vi "FTW-Publisher-Publish.vi"(0 "FTW-Publisher In":refnum<class "FTW-Publisher.lvclass">, 5 "Header":string, 7 "Body":string, 11 "error in":errorcluster) -> (4 "FTW-Publisher Out":refnum<class "FTW-Publisher.lvclass">, 15 "error out":errorcluster)   [LabVIEW 2013, in "FTW-Publisher.lvclass"]
uses:
  FTW-Publisher.lvclass
  Message/Base/FTW-Message.lvclass
  FTW-Publisher.lvclass/FTW-Publisher.ctl
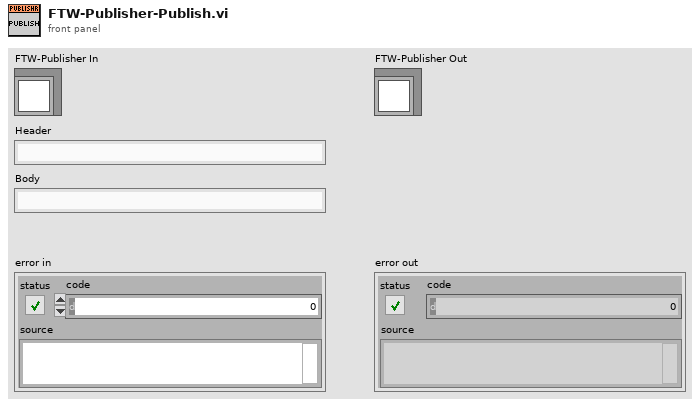
[diagram p1: front panel]
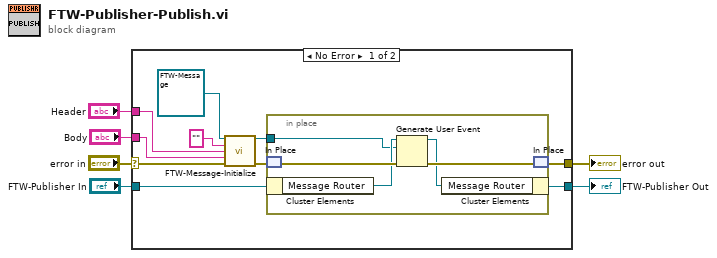
[diagram p0: block diagram]
diagram:
  n1 = case shown="No Error" "error in" {
    selector: "error in" -> [w14 w23]
    tunnel: [w13 w23] -> w3
    tunnel: [w15 w22] -> w5
    tunnel: "FTW-Publisher In" -> [w16 w22]
    tunnel: "Header" -> [w9 _]
    tunnel: "Body" -> [w8 _]
    frame No Error {
      n2 = call-dynamic "FTW-Message-Initialize.vi"("FTW Message"=refnum<class "FTW-Message.lvclass"> refnum, "Sender Identity"="", "Message Header"=w9, "Message Body"=w8, "error in"=w14) -> ("FTW Message out"=w11:refnum<class "FTW-Message.lvclass">, "error out"=w12:errorcluster)  [unwired: 9 in]
      n3 = in-place {
        in-place-border: w11 -> [w17]
        n4 = in-place-match #1(w12) -> (w21:errorcluster)
        n5 = in-place-cluster #2(w16) -> ("Message Router"=w20:refnum<user-event>)
        n6 = Generate User Event(user event=w20, event data cluster=w17, error in=w21) -> (user event out=w18:refnum<user-event>, error out=w19:errorcluster)  [unwired: 1 in]
        n7 = in-place-cluster #2("Message Router"=w18) -> (w15:refnum<class "FTW-Publisher.lvclass">)
        n8 = in-place-match #1(w19) -> (w13:errorcluster)
      }
    }
    frame Error {
    }
  }
  "FTW-Publisher Out" <- w5
  "error out" <- w3
